vi "structsgen.vi"() -> ()   [LabVIEW 2013]
panel:
  in  "types":string[](array[string])=["double", "float", "int64", "int32", "int16", "int8", "uInt64", "uInt32", "uInt16", "uInt8", "LVBoolean", "LStrHandle"]
  out "lvDataCluster.h":string
  in  "names":string[](array[string])=["Double", "Single", "I64", "I32", "I16", "I8", "U64", "U32", "U16", "U8", "Boolean", "String"]
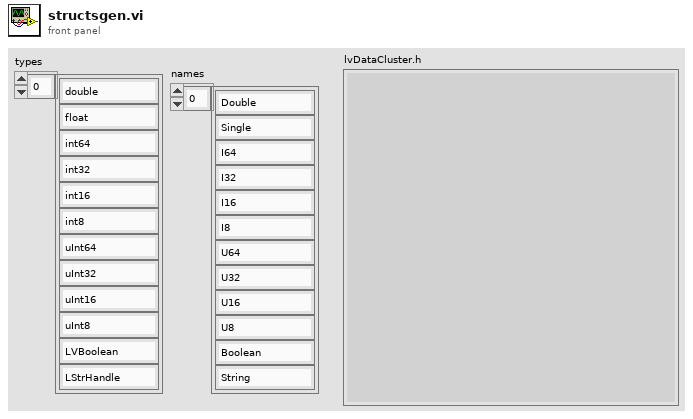
[diagram p1: front panel]
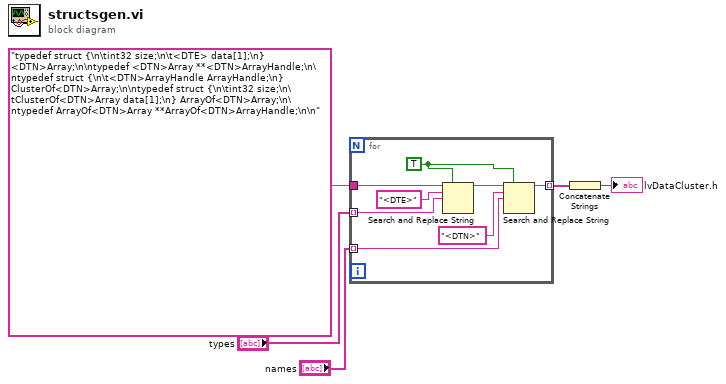
[diagram p0: block diagram]
diagram:
  n1 = for {
    tunnel: "types" -> [w7] mode=indexing
    tunnel: "names" -> [w9] mode=indexing
    tunnel: "typedef struct {\n\tint32 size;\n\t<DTE> data[1];\n} <DTN>Array;\n\ntypedef <DTN>Array **<DTN>ArrayHandle;\n\ntypedef struct {\n\t<DTN>ArrayHandle ArrayHandle;\n} ClusterOf<DTN>Array;\n\ntypedef struct {\n\tint32 size;\n\tClusterOf<DTN>Array data[1];\n} ArrayOf<DTN>Array;\n\ntypedef ArrayOf<DTN>Array **ArrayOf<DTN>ArrayHandle;\n\n" -> [w13]
    tunnel: [w11] -> w3 mode=indexing
    w6 = TRUE ("replace all? (F)")
    n2 = Search and Replace String(replace all?=w6, input string=w13, search string="<DTE>", replace string=w7) -> (result string=w12:string)  [unwired: 4 in, 3 out]
    n3 = Search and Replace String(replace all?=w6, input string=w12, search string="<DTN>", replace string=w9) -> (result string=w11:string)  [unwired: 4 in, 3 out]
  }
  n4 = Concatenate Strings(w3) -> (→"lvDataCluster.h":string)
